vi "Destroy.vi"(8 "error in (no error)":errorcluster, 11 "LV DEV in":refnum<class "LV DEV.lvclass">) -> (0 "error out":errorcluster, 3 "LV DEV out":refnum<class "LV DEV.lvclass">)   [LabVIEW 2016, in "LV DEV.lvclass"]
uses:
  LV DEV.lvclass
  LV Doc.lvclass
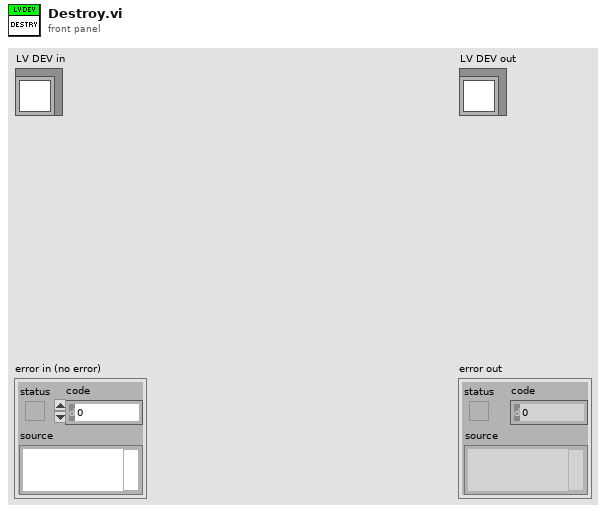
[diagram p1: front panel]
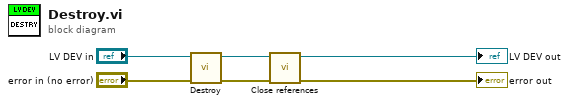
[diagram p0: block diagram]
diagram:
  n1 = call-parent "Destroy.vi"("error in (no error)"="error in (no error)", "Document in"="LV DEV in") -> ("error out"=w2:errorcluster, "Document out"=w4:refnum<class "LV DEV.lvclass">)  [unwired: 8 in]
  n2 = call-dynamic "Close references.vi"("LV DEV in"=w4, "error in (no error)"=w2) -> ("LV DEV out"=→"LV DEV out":refnum<class "LV DEV.lvclass">, "error out"=→"error out":errorcluster)  [unwired: 12 in]
